vi "Fetch Measurement (N Cycle Jitter).vi"(0 "VISA resource name":refnum<visa-resource-name>, 1 "Number Cycle (5)":i32=5 format="%.0g", 2 "Start Cycle (1)":i32=1 format="%.0g", 5 "Channel (1: Channel 1)":i32(ring)=1 items=["Channel 1"=1, "Channel 2"=2, "Channel 3"=3, "Channel 4"=4, "Function 1"=5, "Function 2"=6, "Function 3"=7, "Function 4"=8, "Memory 1"=9, "Memory 2"=10, "Memory 3"=11, "Memory 4"=12], 7 "Edge (0: Rising)":i32(ring) items=["Rising", "Falling"], 11 "error in (no error)":errorcluster) -> (4 "VISA resource name out":refnum<visa-resource-name>, 6 "N cycle jitter (s)":dbl, 15 "error out":errorcluster)   [LabVIEW 2012, in "Agilent 8000 Series.lvlib"]
doc: "Obtains a waveform measurement(N Cycle Jitter) and returns the measurement value. The waveform on which the oscilloscope calculates the waveform measurement is from an acquisition that you previously initiated. \n\nUse the Initiate Acquisition.vi to start an acquisition on the channels that you enable with the Configure Channel.vi. The oscilloscope acquires waveforms for the enabled channels concurrently. You use the Wait For Operation Complete.vi to wait for operation complete. You call this VI separately for each waveform measurement you want to obtain on a specific channel.\n\nYou can call the Read Measurement.vi instead of the Initiate Acquisition.vi. The Read Measurement.vi starts an acquisition on all enabled channels. It then waits for the acquisition to complete, obtains a waveform measurement on the channel you specify, and returns the measurement value. You call this VI separately for any other waveform measurement that you want to obtain on a specific channel.\n\nNotes:\n\n(1) You must configure the appropriate reference levels before you call this VI to take measurement.\n\n(2) You configure the low, mid, and high references either by calling the Configure Reference Levels.vi.\n\n(3) This VI does not check the instrument status. Typically, you call this VI only in a sequence of calls to other low-level driver VIs. The sequence performs one operation. You use the low-level VIs to optimize one or more aspects of interaction with the instrument. If you want to check the instrument status, call the Error-Query.vi at the conclusion of the sequence."
uses:
  Agilent 8000 Series.lvlib
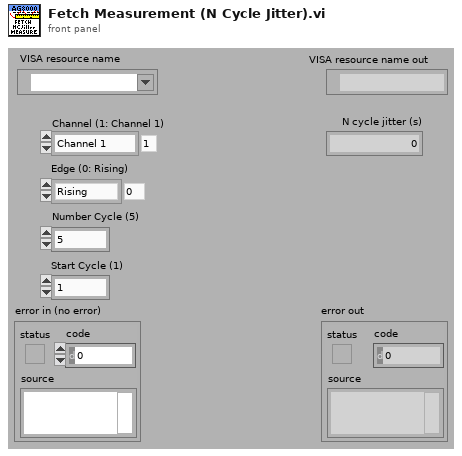
[diagram p1: front panel]
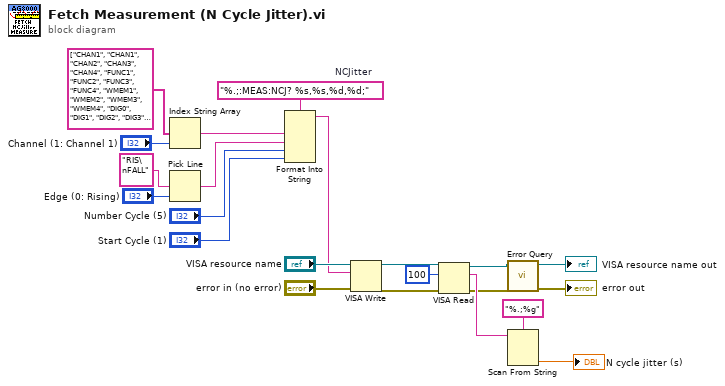
[diagram p0: block diagram]
diagram:
  w17 = "%.;:MEAS:NCJ? %s,%s,%d,%d;"  # NCJitter
  n1 = Index String Array(1:"Channel (1: Channel 1)", 2:string[] ["CHAN1", "CHAN1", "CHAN2", "CHAN3", "CHAN4", "FUNC1", "FUNC2", "FUNC3", "FUNC4", "WMEM1", "WMEM2", "WMEM3", "WMEM4", "DIG0", "DIG1", "DIG2", "DIG3", "DIG4", "DIG5", "DIG6", "DIG7", "DIG8", "DIG9", "DIG10", "DIG11", "DIG12", "DIG13", "DIG14", "DIG15", "AUX", "LINE"]) -> (0:w16:string)  [unwired: 1 in]
  n2 = Pick Line(multi-line string="RIS\nFALL", line index="Edge (0: Rising)") -> (output string=w14:string)  [unwired: 1 in]
  n3 = Format Into String(format string=w17, w16, w14, "Number Cycle (5)", "Start Cycle (1)") -> (resulting string=w9:string)  [unwired: 2 in, 1 out]
  n4 = VISA Write(VISA resource name="VISA resource name", write buffer=w9, error in (no error)="error in (no error)") -> (VISA resource name out=w5:refnum<visa-resource-name>, error out=w4:errorcluster)  [unwired: 1 out]
  n5 = VISA Read(VISA resource name=w5, byte count=u32 100, error in (no error)=w4) -> (VISA resource name out=w3:refnum<visa-resource-name>, read buffer=w7:string, error out=w1:errorcluster)  [unwired: 1 out]
  n6 = call "Error Query.vi"("error in (no error)"=w1, "VISA resource name"=w3) -> ("error out"=→"error out":errorcluster, "VISA resource name out"=→"VISA resource name out":refnum<visa-resource-name>)  [unwired: 6 in, 2 out]
  n7 = Scan From String(format string="%.;%g", input string=w7) -> (output 1=→"N cycle jitter (s)":dbl)  [unwired: 3 in, 3 out]
